vi "Build String.vi"(7 "Section":string[](array[string]), 8 "error in (no error)":errorcluster, 9 "Content":T1[](array[typedef]), 10 "Keys":string[](array[string]), 11 "ConfigManager.Text in":refnum<class "ConfigManager.Text.INI.lvclass">) -> (0 "error out":errorcluster, 2 "Input String":string, 3 "ConfigManager.Text out":refnum<class "ConfigManager.Text.INI.lvclass">)   [LabVIEW 2013, in "CfgManager.Text.lvlib" / "ConfigManager.Text.INI.lvclass"]
uses:
  ConfigManager.Text.INI.lvclass
  Manager.Text/Dictionary Payload -- cluster.ctl
  Manager.Text/ConfigManager.Text.lvclass/ConfigManager.Text.ctl
  Manager.Text/ConfigManager.Text.lvclass
  <vilib>/LabVIEW Open Source Project/Unicity/Delimiter/Delimiter.lvclass
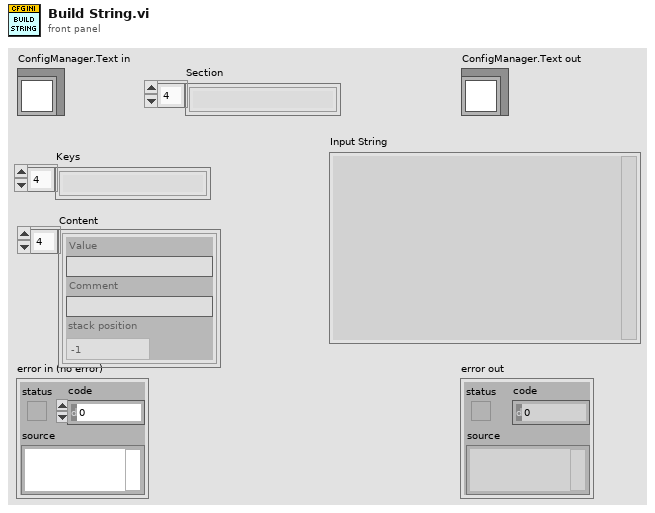
[diagram p1: front panel]
types:
  T1 = typedef "CfgManager.Text.lvlib/ConfigManager.Text.lvclass/Dictionary Payload -- cluster.ctl" = cluster{"Value":string, "Comment":string, "stack position":i32}
  T2 = cluster{"stack position":i32, "Section":string, "key":string, "Content":T1}
  T3 = cluster{"stack position":i32, "Section":string, "key":string, "Content":T1}[]
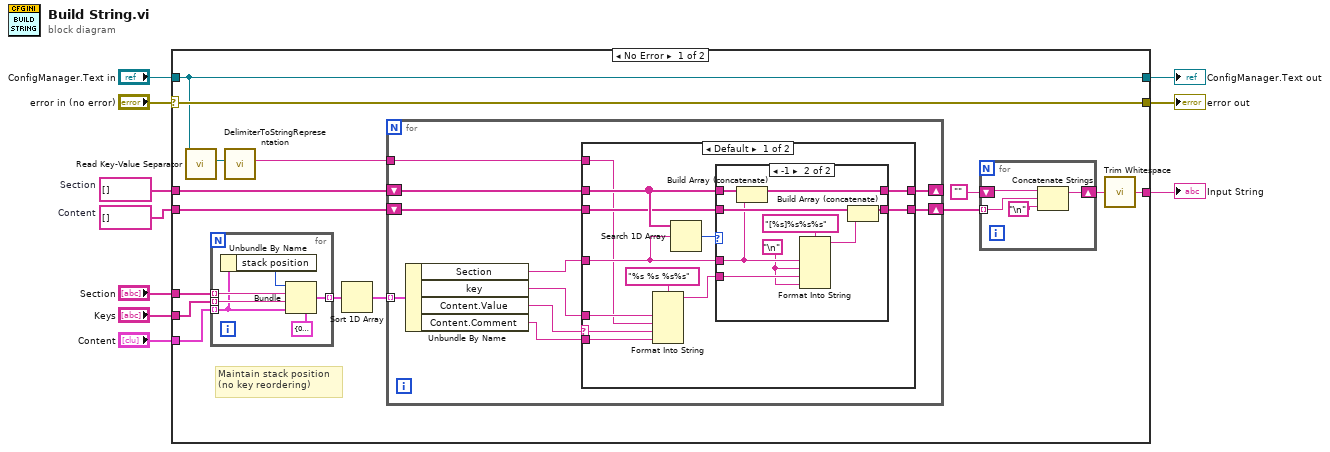
[diagram p0: block diagram]
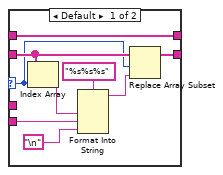
[diagram p2: hidden frame]
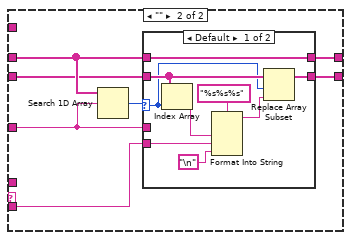
[diagram p3: hidden frame]
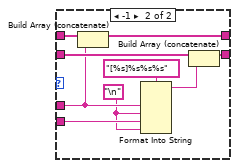
[diagram p4: hidden frame]
diagram:
  w1 = string[] []  # Content
  w2 = string[] []  # Section
  n1 = case shown="No Error" "error in (no error)" {
    selector: "error in (no error)" -> [w25 w102]
    tunnel: [w25 w102] -> w9
    tunnel: [w22 w101] -> w7
    tunnel: "ConfigManager.Text in" -> [w22 w101]
    tunnel: "Section" -> [w13 _]
    tunnel: "Keys" -> [w14 _]
    tunnel: "Content" -> [w15 _]
    tunnel: [w16 _] -> w3
    tunnel: w2 -> [w24 _]
    tunnel: w1 -> [w23 _]
    frame No Error {
      # "Maintain stack position\n(no key reordering)"
      n2 = call "Read Key-Value Separator.vi"("ConfigManager.Text in"=w22) -> ("Key Value Separator"=w21:refnum<class "Delimiter.lvclass">)  [unwired: 9 in, 1 out]
      n3 = for {
        tunnel: w15 -> [w28] mode=indexing
        tunnel: w14 -> [w29] mode=indexing
        tunnel: w13 -> [w30] mode=indexing
        tunnel: [w27] -> w12 mode=indexing
        n4 = Unbundle By Name(w28) -> ("stack position"=w31:i32)
        n5 = Bundle(cluster=T2 {"stack position"=0, "Section"="", "key"="", "Content"={"Value"="", "Comment"="", "stack position"=0}}, "stack position"=w31, "Section"=w30, "key"=w29, "Content"=w28) -> (w27:T2)
      }
      n6 = call <vilib>:"DelimiterToStringRepresentation.vi"("Delimiter"=w21) -> ("String representation"=w20:string)  [unwired: 10 in]
      n7 = Sort 1D Array(array=w12) -> (sorted array=w11:T3)
      n8 = for {
        shift-right: [w43] -> _
        shift-left: w24 -> [w45]
        shift-right: [w42] -> w19
        shift-left: w23 -> [w44]
        tunnel: w20 -> [w41]
        tunnel: w11 -> [w39] mode=indexing
        n9 = Unbundle By Name(w39) -> ("Section"=w40:string, "key"=w38:string, "Content.Value"=w37:string, "Content.Comment"=w36:string)
        n10 = case shown="Default" w37 {
          selector: w37 -> [w49 _]
          tunnel: w45 -> [w56 w81]
          tunnel: w40 -> [w55 w80]
          tunnel: w44 -> [w54 w79]
          tunnel: w38 -> [w53 _]
          tunnel: [w52 w78] -> w43
          tunnel: [w51 w77] -> w42
          tunnel: w41 -> [w50 _]
          tunnel: w36 -> [w48 w76]
          frame Default {
            n11 = Format Into String(format string="%s %s %s%s", w53, w50, w49, w48) -> (resulting string=w46:string)  [unwired: 2 in, 1 out]
            n12 = Search 1D Array(1D array=w56, element=w55) -> (index of element=w57:i32)  [unwired: 1 in]
            n13 = case shown="-1" w57 {
              selector: w57 -> [w60 _]
              tunnel: w56 -> [w66 w75]
              tunnel: w55 -> [_ w71]
              tunnel: w54 -> [w65 w73]
              tunnel: w46 -> [w59 w70]
              tunnel: [w66 w74] -> w52
              tunnel: [w64 w72] -> w51
              frame Default {
                n14 = Index Array(array=w65, index=w60) -> (element=w63:string)
                n15 = Format Into String(format string="%s%s%s", w63, w59, "\n") -> (resulting string=w61:string)  [unwired: 2 in, 1 out]
                n16 = Replace Array Subset(array=w65, new element=w61, index=w60) -> (w64:string[])
              }
              frame -1 {
                w67 = "\n"
                n17 = Build Array (concatenate)(w75, w71) -> (w74:string[])
                n18 = Format Into String(format string="[%s]%s%s%s", w71, w67, w70, w67) -> (resulting string=w69:string)  [unwired: 2 in, 1 out]
                n19 = Build Array (concatenate)(w73, w69) -> (w72:string[])
              }
            }
          }
          frame "" {
            n20 = Search 1D Array(1D array=w81, element=w80) -> (index of element=w82:i32)  [unwired: 1 in]
            n21 = case shown="Default" w82 {
              selector: w82 -> [w85 _]
              tunnel: w81 -> [w91 w100]
              tunnel: w80 -> [_ w96]
              tunnel: w79 -> [w90 w98]
              tunnel: w76 -> [w84 w95]
              tunnel: [w91 w99] -> w78
              tunnel: [w89 w97] -> w77
              frame Default {
                n22 = Index Array(array=w90, index=w85) -> (element=w88:string)
                n23 = Format Into String(format string="%s%s%s", w88, w84, "\n") -> (resulting string=w86:string)  [unwired: 2 in, 1 out]
                n24 = Replace Array Subset(array=w90, new element=w86, index=w85) -> (w89:string[])
              }
              frame -1 {
                w92 = "\n"
                n25 = Build Array (concatenate)(w100, w96) -> (w99:string[])
                n26 = Format Into String(format string="[%s]%s%s%s", w96, w92, w95, w92) -> (resulting string=w94:string)  [unwired: 2 in, 1 out]
                n27 = Build Array (concatenate)(w98, w94) -> (w97:string[])
              }
            }
          }
        }
      }
      n28 = for {
        tunnel: w19 -> [w34] mode=indexing
        shift-right: [w32] -> w17
        shift-left: "" -> [w35]
        n29 = Concatenate Strings(w35, w34, "\n") -> (w32:string)
      }
      n30 = call <vilib>:"Trim Whitespace.vi"("string"=w17) -> ("trimmed string"=w16:string)  [unwired: 1 in]
    }
    frame Error {
    }
  }
  "error out" <- w9
  "ConfigManager.Text out" <- w7
  "Input String" <- w3
